vi "Error_ReadMsgRef.vi"(6 "error in (no error)":errorcluster, 9 "vi path":path) -> (0 "error out":errorcluster, 2 "ErrorMsgArray":refnum<vi>, 3 "ErrorMsg":refnum<vi>)   [LabVIEW 2016]
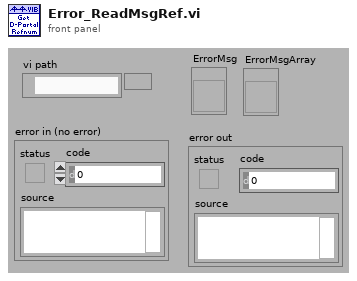
[diagram p1: front panel]
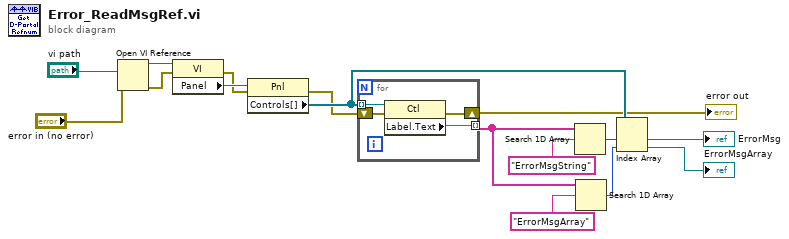
[diagram p0: block diagram]
diagram:
  n1 = Open VI Reference(vi path="vi path", error in (no error)="error in (no error)") -> (vi reference=w15:refnum<vi>, error out=w8:errorcluster)  [unwired: 4 out]
  n2 = property class="VI"(reference=w15, error in=w8) -> (error out=w9:errorcluster, "Panel"=w10:refnum<vi>)  [unwired: 1 out]
  n3 = property class="Pnl"(reference=w10, error in=w9) -> (error out=w11:errorcluster, "Controls[]"=w12:refnum<vi>[])  [unwired: 1 out]
  n4 = for {
    tunnel: w12 -> [w20] mode=indexing
    tunnel: [w19] -> w3 mode=indexing
    shift-right: [w17] -> w5
    shift-left: w11 -> [w18]
    n5 = property class="Ctl"(reference=w20, error in=w18) -> (error out=w17:errorcluster, "Label.Text"=w19:string)  [unwired: 1 out]
  }
  "error out" <- w5
  n6 = Search 1D Array(1D array=w3, element="ErrorMsgString") -> (index of element=w13:i32)  [unwired: 1 out]
  n7 = Search 1D Array(1D array=w3, element="ErrorMsgArray") -> (index of element=w1:i32)  [unwired: 1 out]
  n8 = Index Array(array=w12, index #1=w13, index #2=w1) -> (element #1=→"ErrorMsg":refnum<vi>, element #2=→"ErrorMsgArray":refnum<vi>)
